vi "FTW-Supervisor-Core-Process.vi"(0 "FTW Supervisor Configuration":string, 11 "error in":errorcluster) -> (15 "error out":errorcluster)   [LabVIEW 2015, in "FTW-Supervisor.lvclass"]
uses:
  FTW-Supervisor.lvclass
  instance/FTW-Actor-Instance.lvclass
  json/FTW-JSON-Type.ctl
  codegen/xnode/FTW-JSON-Fetch.xnode
  core/type/FTW-Type-JSON.ctl
  lib/FTW-KernelFilepath.vi
  json/core/FTW-JSON-Core-LibraryReturnValue.vi
  error/FTW-ERR-ThrowInvalidReferenceError.vi
  json/core/FTW-JSON-Core-Type.ctl
  json/core/FTW-JSON-Core-ElementType.vi
panel:
  # "Inputs"
  # "Outputs"
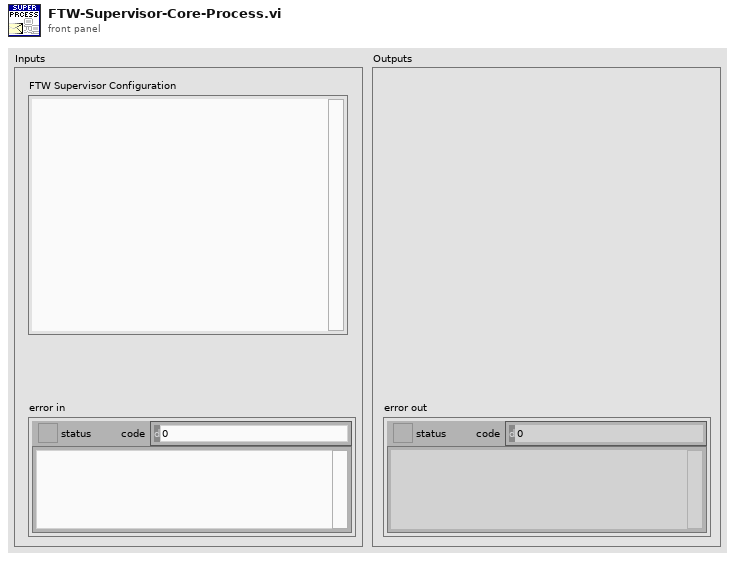
[diagram p1: front panel]
types:
  T1 = typedef "FTW-JSON-Core-Type.ctl" = enum8{"Object", "Array", "String", "Integer", "Floating Point", "true", "false", "null", "undefined"}
  T2 = typedef "FTW-Type-JSON.ctl" = refnum<data-value>
  T3 = typedef "FTW-Type-SQLite.ctl" = refnum<data-value>
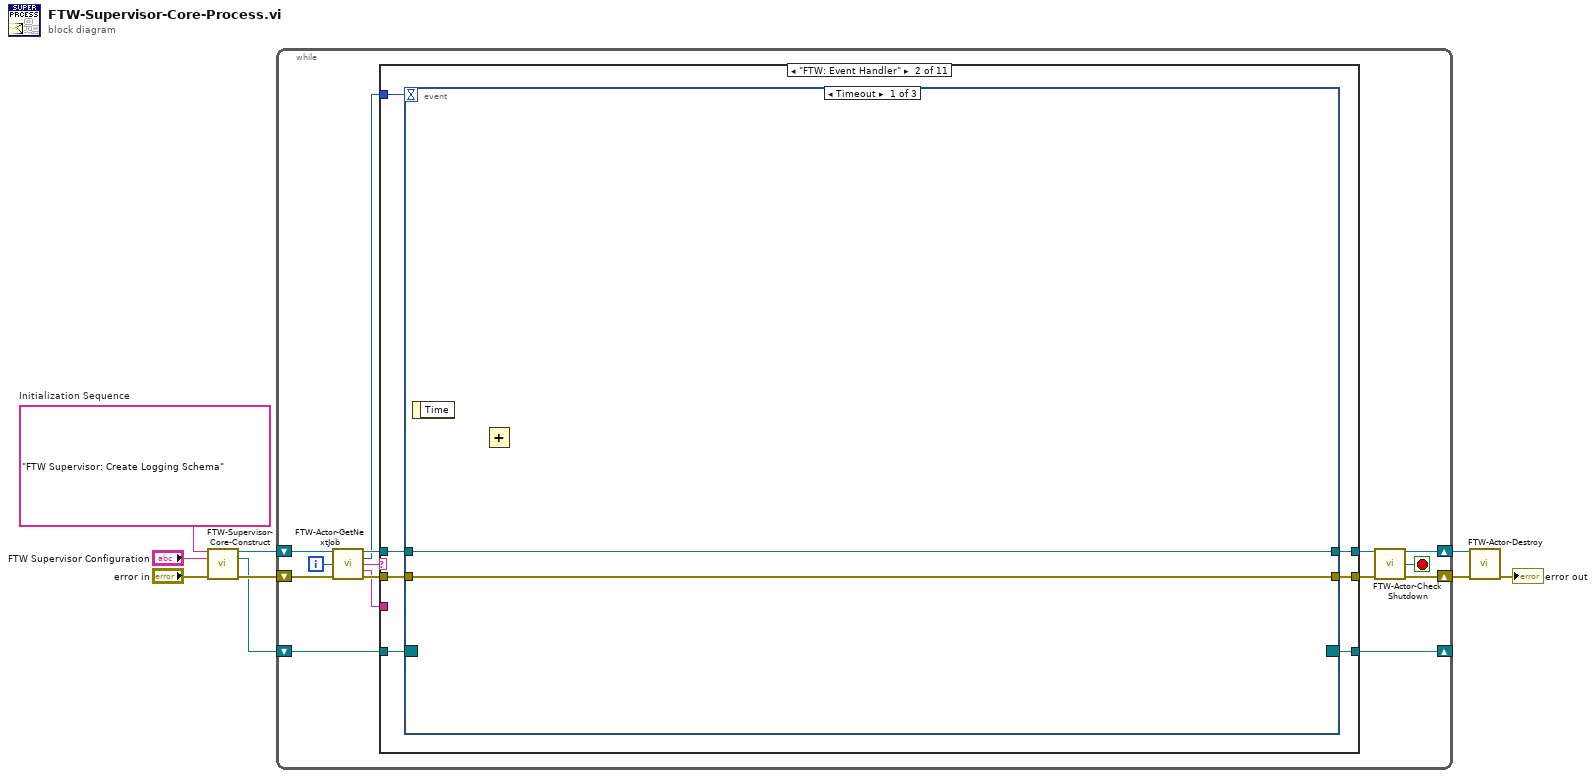
[diagram p0: block diagram]
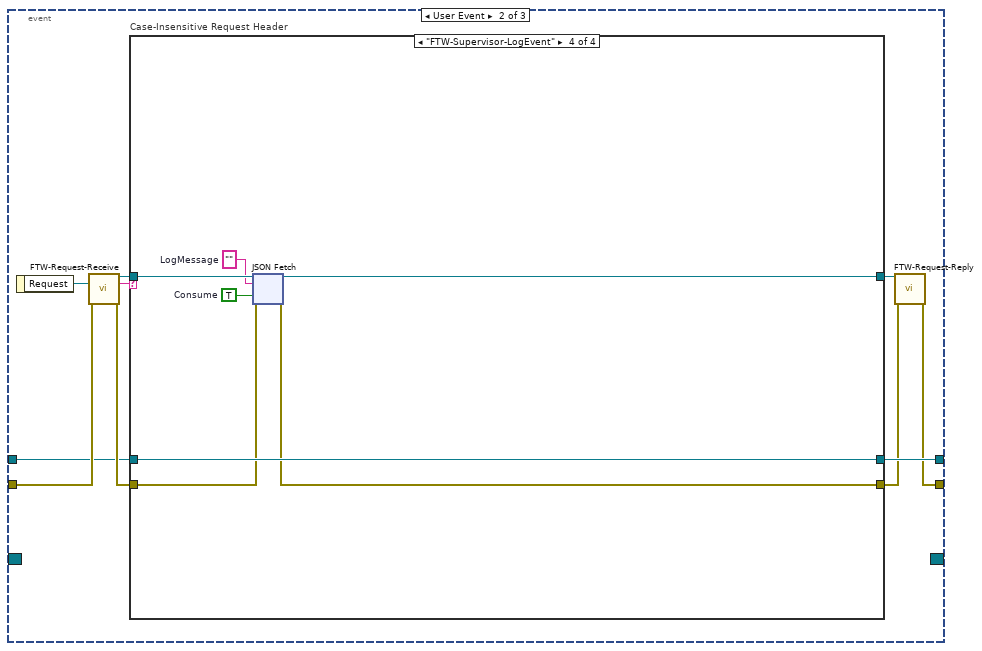
[diagram p3: hidden frame]
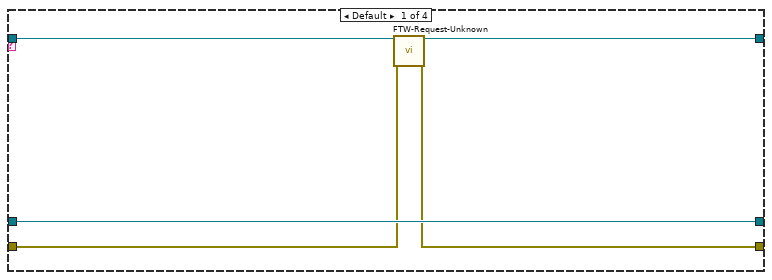
[diagram p4: hidden frame]
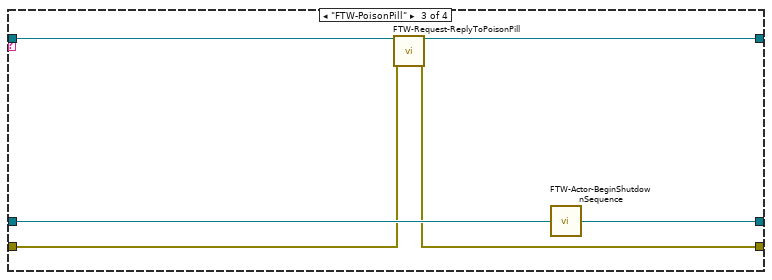
[diagram p6: hidden frame]
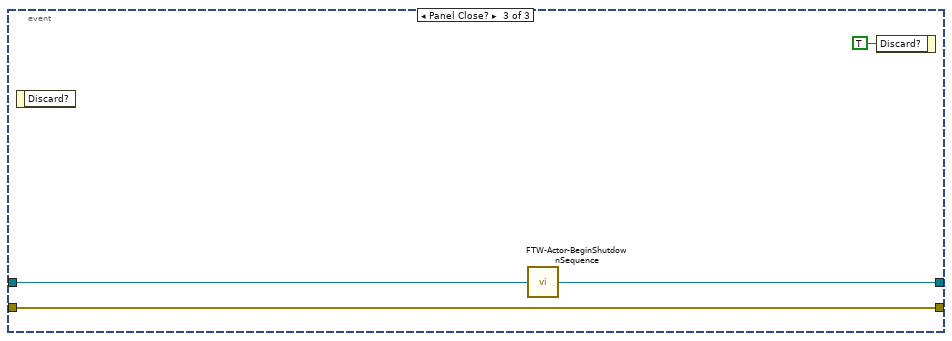
[diagram p7: hidden frame]
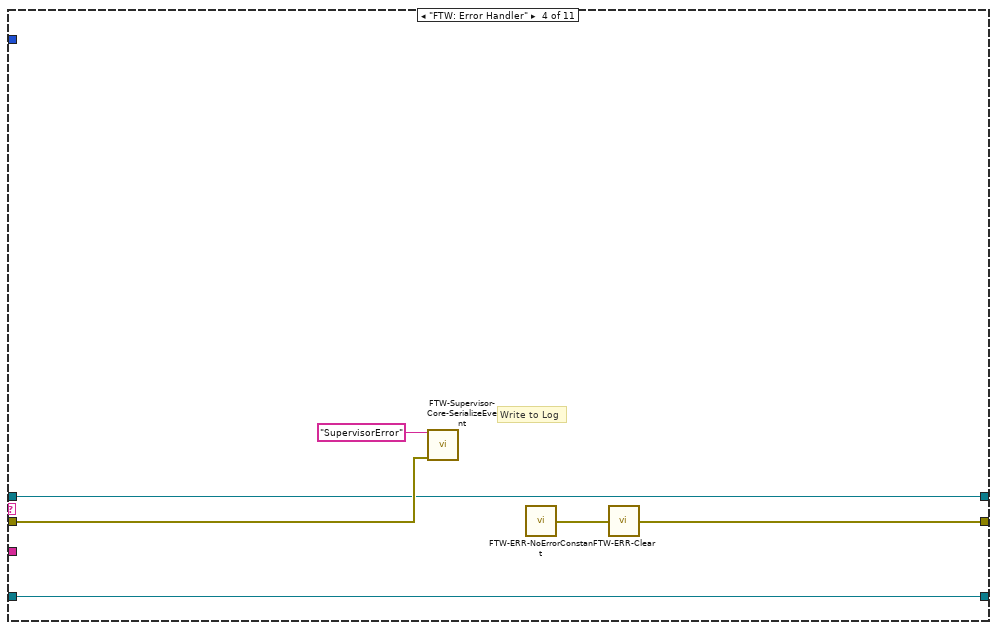
[diagram p9: hidden frame]
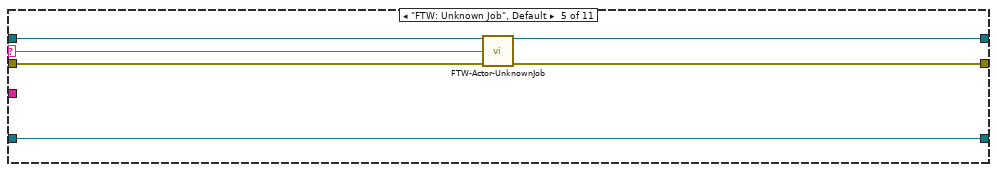
[diagram p10: hidden frame]
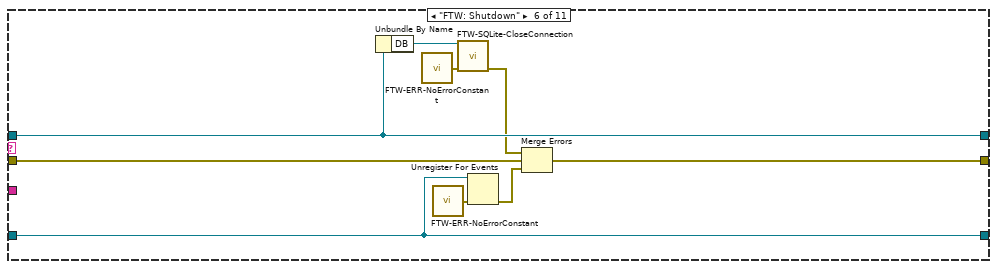
[diagram p11: hidden frame]
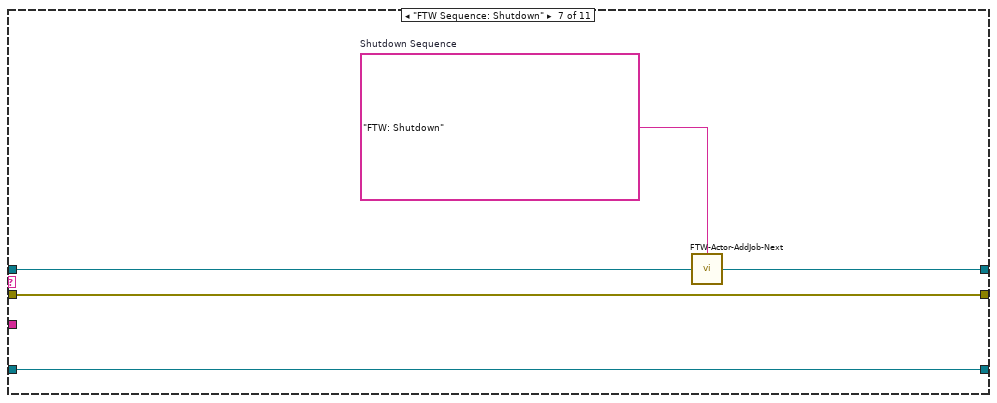
[diagram p12: hidden frame]
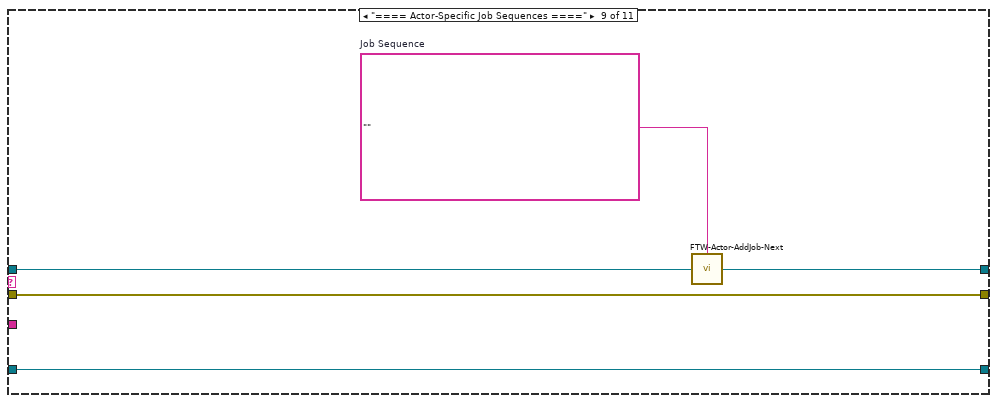
[diagram p14: hidden frame]
diagram:
  w3 = "FTW Supervisor: Create Logging Schema"  # Initialization Sequence
  n1 = call "FTW-Supervisor-Core-Construct.vi"("Initialization Sequence"=w3, "FTW Supervisor Configuration"="FTW Supervisor Configuration", "error in"="error in") -> ("FTW Supervisor"=w6:refnum<class "FTW-Supervisor.lvclass">, "Incoming Request"=w1:refnum<event-registration>, "error out"=w5:errorcluster)  [unwired: 10 in]
  n2 = while {
    shift-right: [w16] -> w8
    shift-left: w5 -> [w22]
    shift-right: [w23] -> _
    shift-left: w1 -> [w24]
    shift-right: [w15] -> w9
    shift-left: w6 -> [w20]
    i -> [w13]
    stop <- w10 stop-if-true
    n3 = call "FTW-Actor-GetNextJob.vi"("FTW Actor Instance"=w20, "Jobs Performed"=w13, "error in"=w22) -> ("FTW Actor Instance out"=w19:refnum<class "FTW-Supervisor.lvclass">, "Event Structure Timeout"=w11:i32, "Job Name"=w14:string, "Job Data"=w12:string, "error out"=w21:errorcluster)  [unwired: 8 in]
    n4 = case shown="\"FTW: Event Handler\"" w14 {
      selector: w14 -> [_ _ _ _ w125 _ _ _ _ _ _]
      tunnel: [w26 w34 w117 w121 w127 w139 w143 w147 w151 w155 w156] -> w17
      tunnel: w21 -> [w26 w33 w117 w122 w126 w136 w143 w147 w151 w155 w156]
      tunnel: w24 -> [w27 w32 w118 w124 w130 w137 w144 w146 w152 w154 w158]
      tunnel: [w27 w31 w118 w124 w130 w137 w144 w146 w152 w154 w158] -> w23
      tunnel: w19 -> [w25 w29 w116 w119 w129 w134 w141 w145 w149 w153 w157]
      tunnel: [w25 w30 w116 w119 w128 w134 w140 w145 w148 w153 w157] -> w18
      tunnel: w11 -> [_ w28 _ _ _ _ _ _ _ _ _]
      tunnel: w12 -> [_ _ _ _ _ _ _ _ _ _ _]
      frame "==== Featherweight Framework Jobs ====" {
      }
      frame "FTW: Event Handler" {
        n5 = event shown="[0] Timeout" {
          selector: w32 -> [_ _ _]
          dyn-events: [_ _ _] -> w31
          timeout: w28 -> [_ _ _]
          tunnel: [w35 w39 w114] -> w34
          tunnel: w33 -> [w35 w45 w114]
          tunnel: [w36 w44 w112] -> w30
          tunnel: w29 -> [w36 w43 w113]
          event Timeout {
            n6 = event-data() -> ()  [unwired: 1 in, 1 out]
            n7 = Add() -> ()  [unwired: 2 in, 1 out]
          }
          event User Event {
            n8 = event-data() -> ("Request"=w37:refnum<queue>)  [unwired: 1 in]
            n9 = call "FTW-Request-Receive.vi"("MessagePipe"=w37, "error in"=w45) -> ("Request"=w41:T2, "Request Header"=w42:string, "error out"=w46:errorcluster)  [unwired: 11 in]
            n10 = case "Case-Insensitive Request Header" shown="\"FTW-Supervisor-LogEvent\"" w42 {
              tunnel: [w48 w52 w55 w63] -> w38
              tunnel: w46 -> [w49 w52 w56 w64]
              tunnel: [w51 w54 w59 w67] -> w44
              tunnel: w43 -> [w51 w54 w60 w67]
              tunnel: w41 -> [w50 w53 w58 w66]
              tunnel: [w47 w53 w57 w65] -> w40
              frame Default {
                n11 = call "FTW-Request-Unknown.vi"("Request"=w50, "error in"=w49) -> ("Request out"=w47:T2, "error out"=w48:errorcluster)  [unwired: 12 in]
              }
              frame "FTW-ActorStatus" {
              }
              frame "FTW-PoisonPill" {
                n12 = call "FTW-Request-ReplyToPoisonPill.vi"("Poison Pill Request"=w58, "error in"=w56) -> ("Poison Pill Response"=w57:T2, "error out"=w55:errorcluster)  [unwired: 12 in]
                n13 = call "FTW-Actor-BeginShutdownSequence.vi"("FTW Actor Instance"=w60) -> ("FTW Actor Instance out"=w59:refnum<class "FTW-Supervisor.lvclass">)  [unwired: 3 in]
              }
              frame "FTW-Supervisor-LogEvent" {
                w61 = TRUE  # Consume
                w62 = ""  # LogMessage
                n14 = xnode "JSON Fetch"("JSON"=w66, "Element Type and Default Value"=w62, "Consume Element"=w61, "error in"=w64) -> ("JSON out"=w65:T2, "error out"=w63:errorcluster)  [unwired: 1 in, 2 out]
              }
            }
            n15 = call "FTW-Request-Reply.vi"("Request"=w40, "error in"=w38) -> ("error out"=w39:errorcluster)  [unwired: 13 in]
          }
          event Panel Close? {
            n16 = event-data() -> ()  [unwired: 1 in, 1 out]
            n17 = call "FTW-Actor-BeginShutdownSequence.vi"("FTW Actor Instance"=w113) -> ("FTW Actor Instance out"=w112:refnum<class "FTW-Supervisor.lvclass">)  [unwired: 3 in]
            n18 = event-data("Discard?"=TRUE) -> ()  [unwired: 1 in, 1 out]
          }
        }
      }
      frame "FTW: Failure to Launch" {
      }
      frame "FTW: Error Handler" {
        # "Write to Log"
        n19 = call "FTW-Supervisor-Core-SerializeEvent.vi"("Event Type"="SupervisorError", "Error to Log"=w122) -> ()  [unwired: 13 in, 1 out]
        n20 = call "FTW-ERR-NoErrorConstant.vi"() -> ("no error"=w120:errorcluster)
        n21 = call "FTW-ERR-Clear.vi"("error to snuff"=w120) -> ("no error"=w121:errorcluster)
      }
      frame "FTW: Unknown Job", Default {
        n22 = call "FTW-Actor-UnknownJob.vi"("FTW Actor Instance"=w129, "Unknown Job"=w125, "error in"=w126) -> ("FTW Actor Instance out"=w128:refnum<class "FTW-Supervisor.lvclass">, "error out"=w127:errorcluster)  [unwired: 11 in]
      }
      frame "FTW: Shutdown" {
        n23 = Unbundle By Name(w134) -> ("DB"=w135:T3)
        n24 = call "FTW-ERR-NoErrorConstant.vi"() -> ("no error"=w133:errorcluster)
        n25 = call "FTW-ERR-NoErrorConstant.vi"() -> ("no error"=w132:errorcluster)
        n26 = call "FTW-SQLite-CloseConnection.vi"("SQLite Connection"=w135, "error in"=w133) -> ("error out"=w131:errorcluster)  [unwired: 13 in]
        n27 = Unregister For Events(event registration refnum=w137, error in=w132) -> (error out=w138:errorcluster)
        n28 = Merge Errors(w131, w136, w138) -> (w139:errorcluster)
      }
      frame "FTW Sequence: Shutdown" {
        w142 = "FTW: Shutdown"  # Shutdown Sequence
        n29 = call "FTW-Actor-AddJob-Next.vi"("Add Next in Job Queue"=w142, "FTW Actor Instance"=w141) -> ("FTW Actor Instance out"=w140:refnum<class "FTW-Supervisor.lvclass">)  [unwired: 2 in]
      }
      frame "==== Actor-Specific Static Dependencies ====" {
      }
      frame "==== Actor-Specific Job Sequences ====" {
        w150 = ""  # Job Sequence
        n30 = call "FTW-Actor-AddJob-Next.vi"("Add Next in Job Queue"=w150, "FTW Actor Instance"=w149) -> ("FTW Actor Instance out"=w148:refnum<class "FTW-Supervisor.lvclass">)  [unwired: 2 in]
      }
      frame "==== Actor-Specific Jobs ====" {
      }
      frame "FTW Supervisor: Create Logging Schema" {
      }
    }
    n31 = call "FTW-Actor-CheckShutdown.vi"("FTW Actor Instance"=w18, "error in"=w17) -> ("FTW Actor Instance out"=w15:refnum<class "FTW-Supervisor.lvclass">, "Shutdown?"=w10:bool, "error out"=w16:errorcluster)  [unwired: 11 in]
  }
  n32 = call "FTW-Actor-Destroy.vi"("FTW Actor Instance"=w9, "error in"=w8) -> ("error out"=→"error out":errorcluster)  [unwired: 12 in, 1 out]
